vi "Reset.vi"(8 "error in (no error)":errorcluster, 11 "VISA resource name":refnum<visa-resource-name>) -> (0 "error out":errorcluster, 3 "VISA resource name out":refnum<visa-resource-name>)   [LabVIEW 2011, in "Ocean Server OS4000.lvlib"]
doc: "Resets the instrument and then sends a set of default setup commands to the instrument."
uses:
  Ocean Server OS4000.lvlib
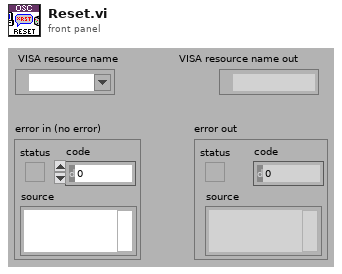
[diagram p1: front panel]
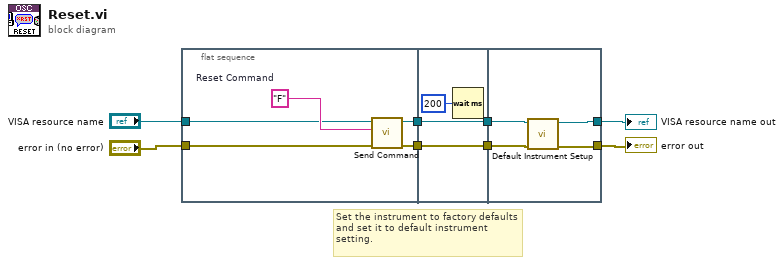
[diagram p0: block diagram]
diagram:
  # "Set the instrument to factory defaults and set it to default instrument setting."
  n1 = flat-sequence {
    tunnel: [w12] -> w6
    tunnel: [w11] -> w4
    tunnel: "VISA resource name" -> [w10]
    tunnel: "error in (no error)" -> [w9]
    tunnel: w6 -> [w16]
    tunnel: [w16] -> w5
    tunnel: w4 -> [w15]
    tunnel: [w15] -> w3
    tunnel: [w19] -> w7
    tunnel: [w17] -> w8
    tunnel: w5 -> [w18]
    tunnel: w3 -> [w20]
    frame #0 {
      w13 = "F"  # Reset Command
      n2 = call "Send Command.vi"("error in (no error)"=w9, "Message"=w13, "VISA resource name"=w10) -> ("error out"=w12:errorcluster, "VISA resource out"=w11:refnum<visa-resource-name>)  [unwired: 7 in]
    }
    frame #1 {
      n3 = Wait (ms)(milliseconds to wait=u32 200) -> ()  [unwired: 1 out]
    }
    frame #2 {
      n4 = call "Default Instrument Setup.vi"("error in (no error)"=w18, "VISA resource name"=w20) -> ("error out"=w17:errorcluster, "VISA resource out"=w19:refnum<visa-resource-name>)  [unwired: 8 in]
    }
  }
  "error out" <- w8
  "VISA resource name out" <- w7
